vi "Process Incoming Messages by PDU F.vi"(8 "error in":errorcluster, 10 "CAN Frame":T1 {"payload" format="%x"; "timestamp" format="%<%.7X\n%x>T"; "type" items=["CAN Data"=0, "CAN Remote"=1, "CAN Bus Error"=2, "J1939 Data"=192, "Delay"=224, "Log Trigger"=225, "Start Trigger"=226]; "identifier" format="%x"}, 11 "internal data":T3={"J1939 XNET Settings"={"XNET Database"="", "XNET Cluster"="", "CAN port"="", "Baud rate [Bd]"=0, "J1939 Network Address"=0, "Name"=0, "Termination"=0}, "j1939 queues"={"Processed Outgoing"=refnum, "Process Outgoing"=refnum, "stop notifier"=refnum, "error queue"=refnum, "active dtc"=refnum, "processed inc"=refnum}, "fgv references"={"BAM Buffer"=refnum, "CM Buffer"=refnum, "CM Gen"=refnum, "BAM Gen"=refnum, "Address Claims"=refnum, "RQST"=refnum, "scaling lut"=refnum, "data lut"=refnum, "cyclic scheduler"=refnum}, "frame in"="", "frame out"="", "timing"={"tb to j1939 queue timeout"=100, "j1939 to tb queue timeout"=100, "dtc loop period (ms)"=100, "CAN in loop period (ms)"=100, "process incoming queue timeout (ms)"=100, "Outgoing Write Decimation"=0, "process outgoing loop rate (ms)"=0, "periodic outgoing queue timeout (ms)"=10, "CAN out queue timeout (ms)"=100}}) -> (0 "error out":errorcluster)   [LabVIEW 2013, in "J1939.lvlib"]
uses:
  J1939.lvlib
  API Types/Internal Data.ctl
  API Types/XNET Settings.ctl
  API Types/Setup Information Cluster.ctl
  API Types/CAN Outgoing Message Cluster.ctl
  API Types/Convert DTCs Cluster.ctl
  <vilib>/xnet/xnet.llb/XNET Frame CAN.ctl
  <vilib>/xnet/xnet.llb/XNET Frame Type CAN.ctl
  TP/TP List References.ctl
  BAM/BAM Buffer Connections List_Ref.ctl
  Connection Mode/Connection Mode Generation Connection Ref.ctl
  BAM/BAM Generation Connections List_Ref.ctl
  LUTs/J1939 Address Table Reference.ctl
  RQST/RQST Lookup Table Reference.ctl
  LUTs/J1939 Conversion Lookup Table Reference.ctl
  LUTs/J1939 Data Lookup Table Reference.ctl
  LUTs/Cyclic Frame Scheduler Lut Reference.ctl
  Configuration/TypeDefs/timing configuration.ctl
  API Types/PGN Fields Cluster.ctl
  TP/TP Connections List State.ctl
  Connection Mode/Connection Mode Buffer Create New TP Connection State.ctl
  LUTs/J1939 Address Lookup Table Action.ctl
  LUTs/J1939 Address Lookup Table Data.ctl
  Frame Conversion/Convert CAN Arb ID to J1939 ID.vi
  Frame Conversion/Convert J1939 ID to CAN Arb ID.vi
  Frame Conversion/Convert CAN Data (U32) to U8.vi
  Common Messages/J1939 Message Acknowledgement.vi
  Buffer Connections List_Actions.vi
  TP/TP Buffer Search for Connection (No PGN).vi
  TP/TP Buffer Add New Data Packet to Connection.vi
  TP/TP Buffer Convert Connection Info to CAN Frame.vi
  TP/TP Buffer Create New TP Connection.vi
  Common Messages/J1939 Message TP.CM EndofMsgACK.vi
  Common Messages/J1939 Message TP.CM CTS.vi
  Common Messages/J1939 Message TP.Conn Abort.vi
  Connection Mode/Connection Mode Generation Connections List_Actions.vi
  Connection Mode/Connection Mode Generation Search for Connection (Remote Message).vi
  TP/TP Buffer Search for Connection.vi
  Connection Mode/Connection Mode Generation CTS Received.vi
  Conversion Lookup Table Get Conversion Parameter.vi
  LUTs/J1939 Data Lookup Table Get Signals (Range).vi
  Frame Conversion/Convert PGN + SA to J1939 ID.vi
  <vilib>/xnet/xnet.llb/XNET Convert.vi
  <vilib>/xnet/xnet.llb/XNET Convert (Signal to Frame Raw).vi
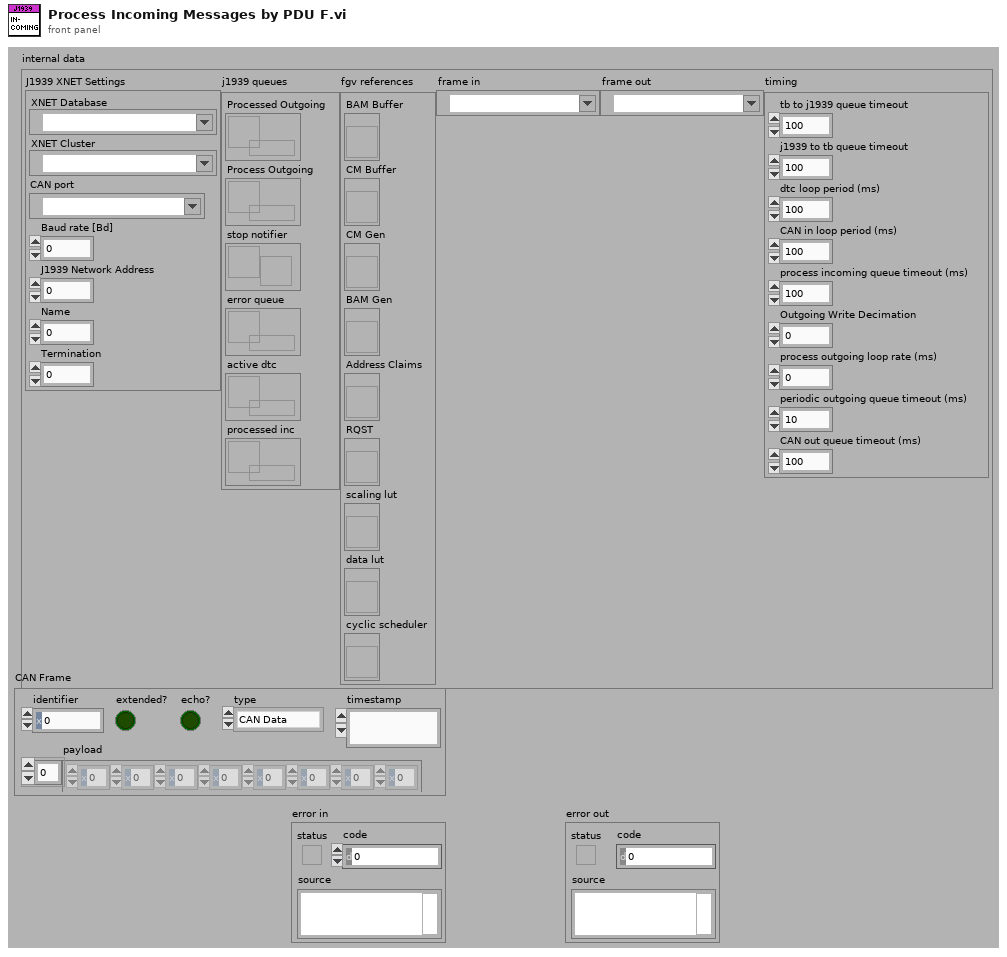
[diagram p1: front panel]
types:
  T1 = typedef "XNET Frame CAN.ctl" = cluster{"timestamp":timestamp, "payload":u8[], "identifier":u32, "type":T2, "extended?":bool, "echo?":bool}
  T2 = typedef "XNET Frame Type CAN.ctl" = u8
  T3 = typedef "J1939.lvlib/Internal Data.ctl" = cluster{"J1939 XNET Settings":T4, "j1939 queues":T5, "fgv references":T6, "frame in":refnum<k21>, "frame out":refnum<k21>, "timing":T15}
  T4 = typedef "J1939.lvlib/XNET settings.ctl" = cluster{"XNET Database":refnum<k21>, "XNET Cluster":refnum<k21>, "CAN port":refnum<k21>, "Baud rate [Bd]":u32, "J1939 Network Address":u8, "Name":u64, "Termination":u32}
  T5 = typedef "J1939.lvlib/Setup Information Cluster.ctl" = cluster{"Processed Outgoing":refnum<queue>, "Process Outgoing":refnum<queue>, "stop notifier":refnum<notifier>, "error queue":refnum<queue>, "active dtc":refnum<queue>, "processed inc":refnum<queue>}
  T6 = typedef "J1939.lvlib/TP List References.ctl" = cluster{"BAM Buffer":T7, "CM Buffer":T7, "CM Gen":T8, "BAM Gen":T9, "Address Claims":T10, "RQST":T11, "scaling lut":T12, "data lut":T13, "cyclic scheduler":T14}
  T7 = typedef "J1939.lvlib/BAM Buffer Connections List_Ref.ctl" = refnum<vi>
  T8 = typedef "J1939.lvlib/Connection Mode Generation Connection Ref.ctl" = refnum<vi>
  T9 = typedef "J1939.lvlib/BAM Generation Connections List_Ref.ctl" = refnum<vi>
  T10 = typedef "J1939.lvlib/J1939 Address Table Reference.ctl" = refnum<vi>
  T11 = typedef "J1939.lvlib/RQST Lookup Table Reference.ctl" = refnum<vi>
  T12 = typedef "J1939.lvlib/J1939 Conversion Lookup Table Reference.ctl" = refnum<vi>
  T13 = typedef "J1939.lvlib/J1939 Data Lookup Table Reference.ctl" = refnum<vi>
  T14 = typedef "J1939.lvlib/cyclic frame scheduler lut reference.ctl" = refnum<vi>
  T15 = typedef "J1939.lvlib/timing configuration.ctl" = cluster{"tb to j1939 queue timeout":i32, "j1939 to tb queue timeout":i32, "dtc loop period (ms)":i32, "CAN in loop period (ms)":i32, "process incoming queue timeout (ms)":i32, "Outgoing Write Decimation":u32, "process outgoing loop rate (ms)":i32, "periodic outgoing queue timeout (ms)":i32, "CAN out queue timeout (ms)":i32}
  T16 = typedef "J1939.lvlib/Message Types.ctl" = enum8{"PDU 1", "RQST2", "XFER", "ACKM", "RQST", "TP.DT - RTS/CTS", "TP.DT - BAM", "TP.CM - RTS", "TP.CM - CTS", "TP.CM - EndofMsgACK", "TP.CM - BAM", "TP.CM - Abort", "TP.CM - Error", "ACL", "Proprietary A", "PDU 2", "Proprietary B", "Error"}
  T17 = typedef "J1939.lvlib/PGN Fields Cluster.ctl" = cluster{"Reserved Bit":u8, "Data page":u8, "PDU Format":u8, "PDU Specific":u8}
  T18 = typedef "J1939.lvlib/CAN Outgoing Message Cluster.ctl" = cluster{"Identifier":u32, "Data":u8[]}
  T19 = typedef "J1939.lvlib/TP Connections List State.ctl" = enum16{"Add", "Update", "Get", "Remove", "Initialize"}
  T20 = typedef "J1939.lvlib/Connection Mode Buffer Create New TP Connection State.ctl" = enum8{"Find Connection", "Create Connection", "Create CTS Frame", "Abort New Connection"}
  T21 = typedef "J1939.lvlib/J1939 Address Lookup Table Data.ctl" = cluster{"Name":u8[], "Address":u8}
  T22 = typedef "J1939.lvlib/J1939 Address Lookup Table Action.ctl" = enum16{"Initialize", "Add", "Get", "Remove", "Get All"}
  T23 = typedef "J1939.lvlib/RQST Lookup Table Cluster.ctl" = cluster{"Response Q":refnum<queue>, "Request PGN":u32}
  T24 = typedef "J1939.lvlib/Convert CAN Data (U8) Cluster.ctl" = cluster{"Byte 1":u8, "Byte 2":u8, "Byte 3":u8, "Byte 4":u8, "Byte 5":u8, "Byte 6":u8, "Byte 7":u8, "Byte 8":u8}
  T25 = typedef "J1939.lvlib/TP Buffer Connection Cluster.ctl" = cluster{"Source Address":u8, "Destination Address":u8, "PGN":u32, "Arb ID":u32, "CAN Conversion Index":u32, "Total Expected Bytes":u16, "Total Expected Packets":u8, "Number of Packets Read":u8, "Start Time":u32, "Packets (U8)":u8[], "Timestamp":timestamp}
  T26 = typedef "J1939.lvlib/Connection Mode Generation Connection Cluster.ctl" = cluster{"Total Packets":u8, "Current Packet to Generate":u8, "Packets":T18[], "Previous Time Stamp":u32, "Total Bytes":u16, "Packet Identifier [PDU S + SA]":u16, "Number of Packets to Generate":u8, "PGN":u32}
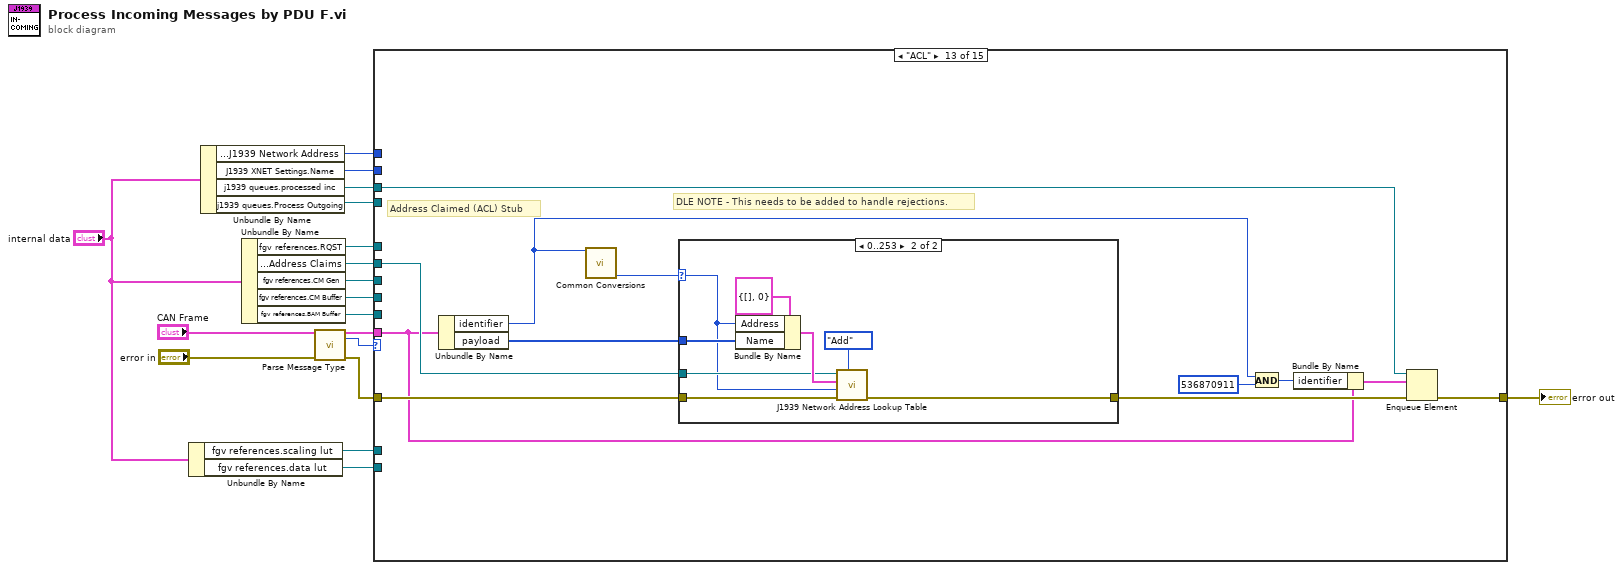
[diagram p0: block diagram]
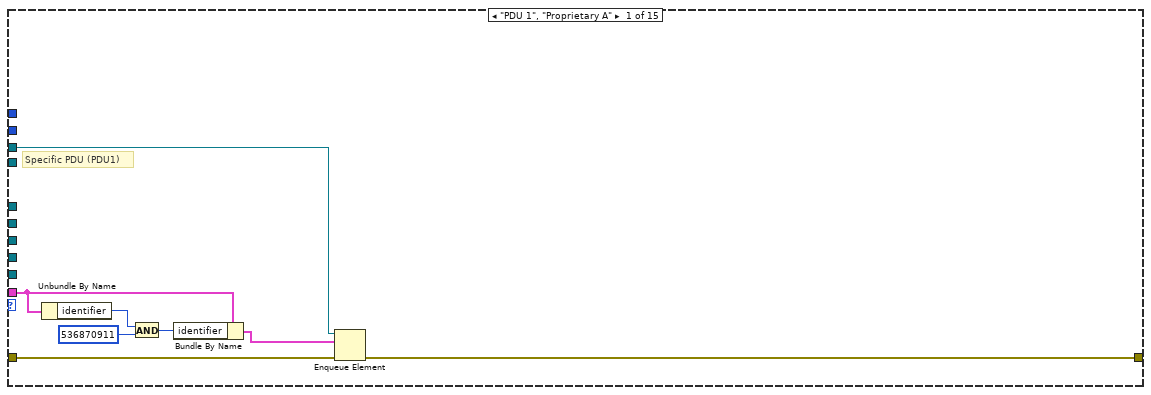
[diagram p2: hidden frame]
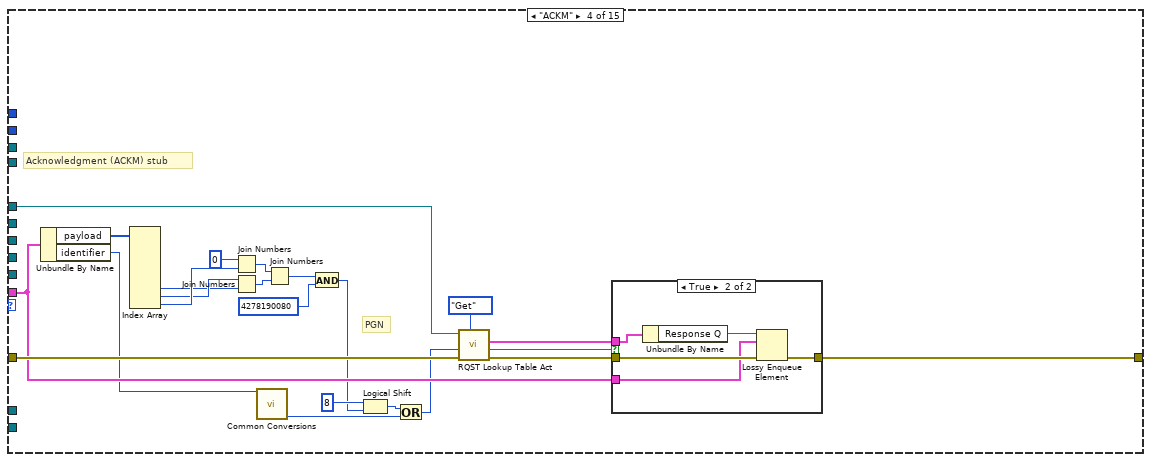
[diagram p5: hidden frame]
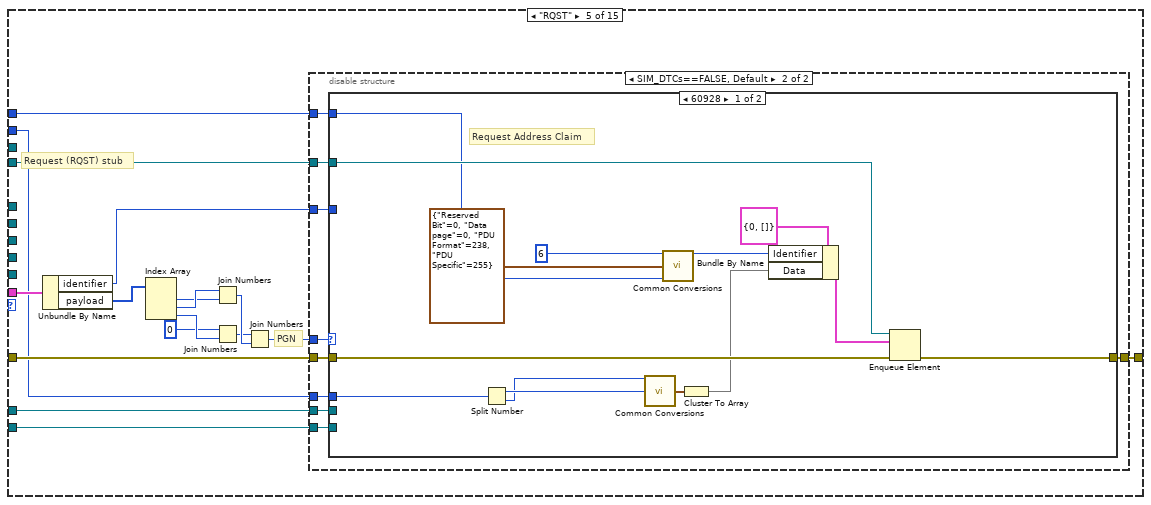
[diagram p7: hidden frame]
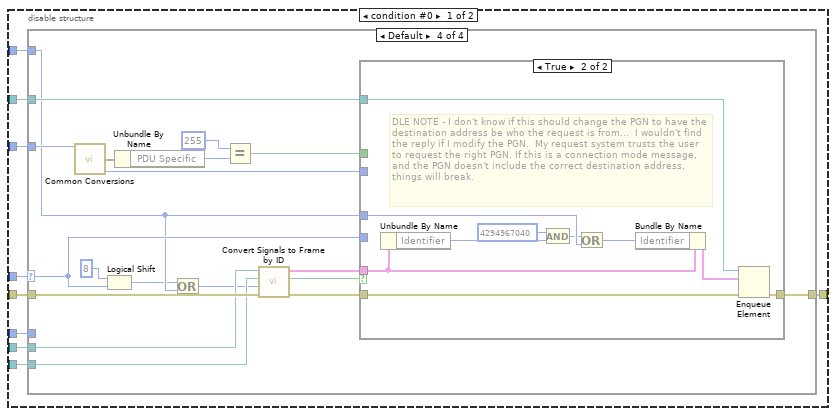
[diagram p8: hidden frame]
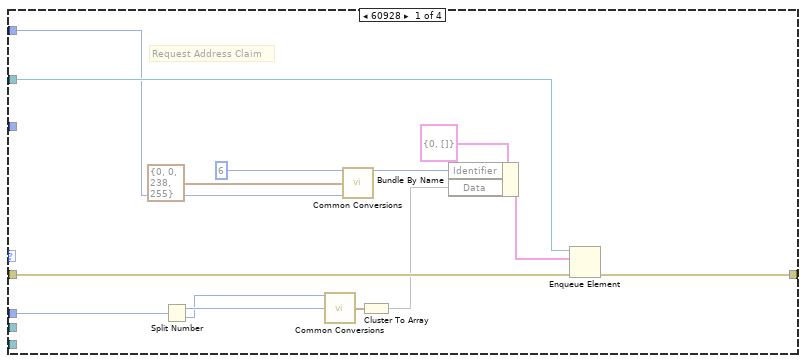
[diagram p9: hidden frame]
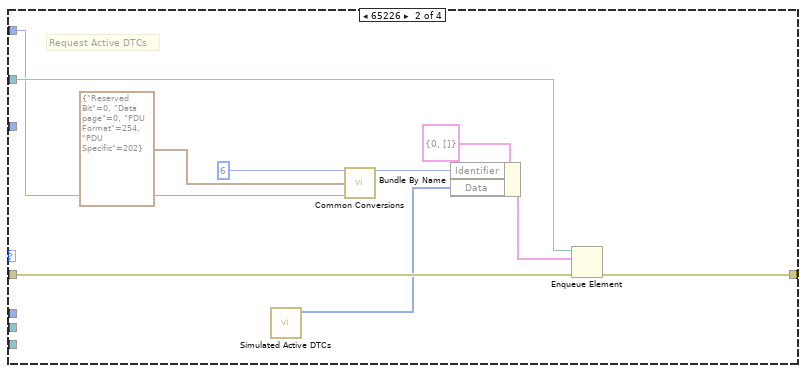
[diagram p10: hidden frame]
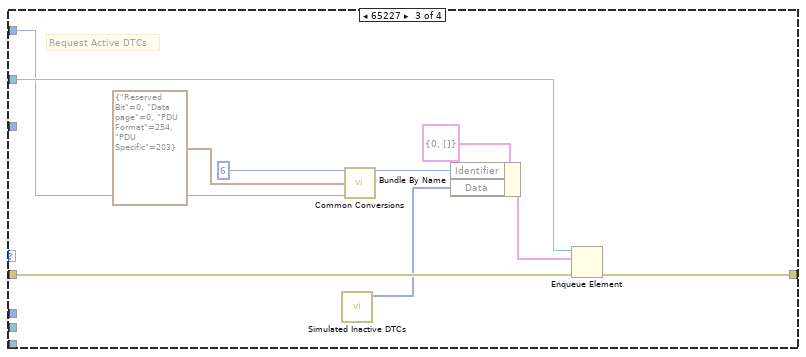
[diagram p11: hidden frame]
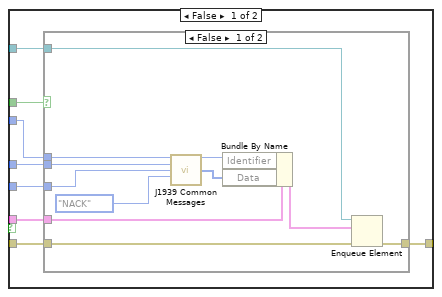
[diagram p12: hidden frame]
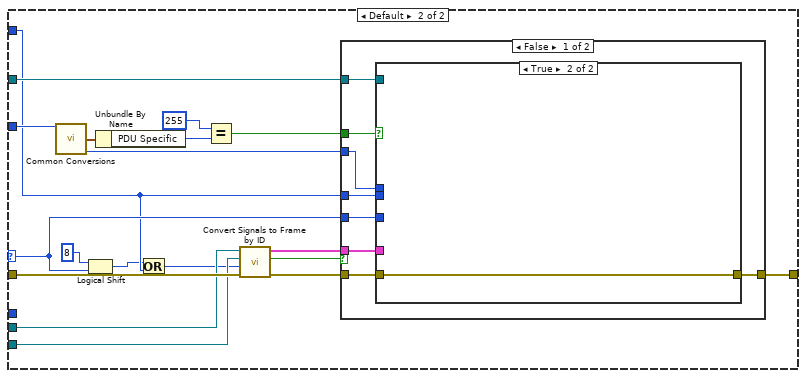
[diagram p14: hidden frame]
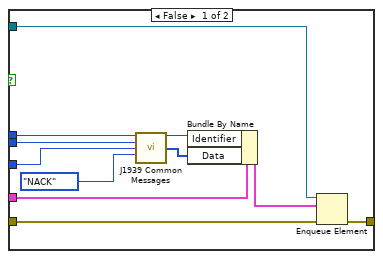
[diagram p15: hidden frame]
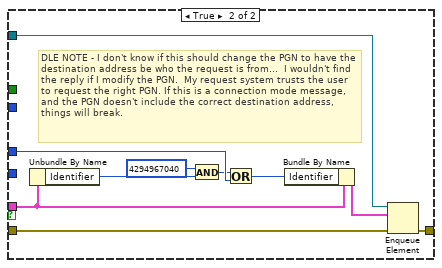
[diagram p16: hidden frame]
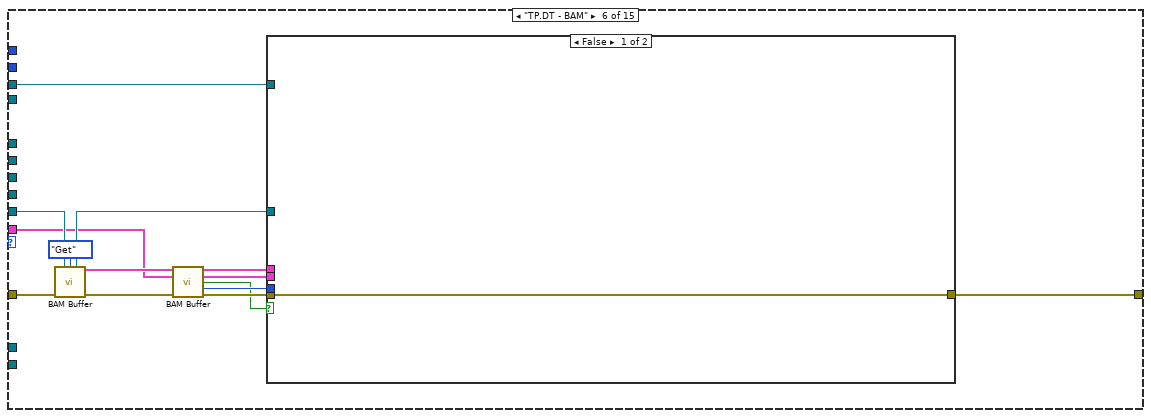
[diagram p17: hidden frame]
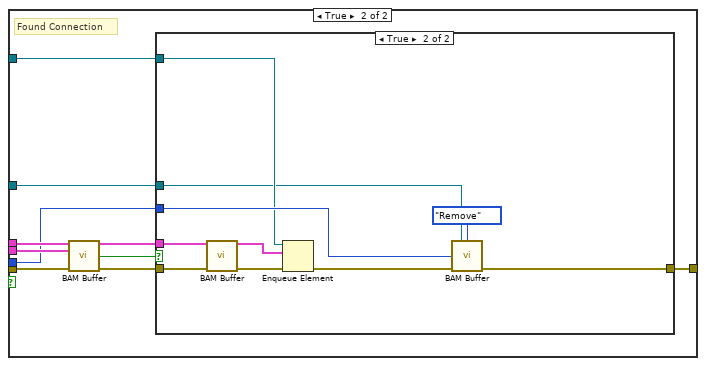
[diagram p18: hidden frame]
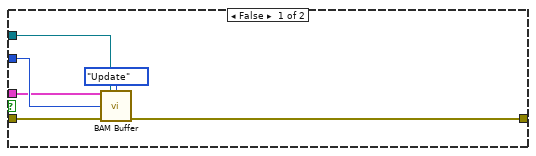
[diagram p19: hidden frame]
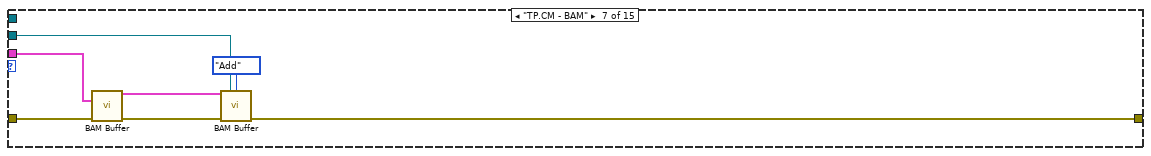
[diagram p20: hidden frame]
diagram:
  n1 = Unbundle By Name("internal data") -> ("fgv references.scaling lut"=w4:T12, "fgv references.data lut"=w3:T13)
  n2 = Unbundle By Name("internal data") -> ("J1939 XNET Settings.J1939 Network Address"=w7:u8, "J1939 XNET Settings.Name"=w8:u64, "j1939 queues.processed inc"=w1:refnum<queue>, "j1939 queues.Process Outgoing"=w13:refnum<queue>)
  n3 = Unbundle By Name("internal data") -> ("fgv references.RQST"=w6:T11, "fgv references.Address Claims"=w9:T10, "fgv references.CM Gen"=w10:T8, "fgv references.CM Buffer"=w11:T7, "fgv references.BAM Buffer"=w12:T7)
  n4 = call "Parse Message Type.vi"("CAN frame"="CAN Frame", "error in"="error in") -> ("CAN frame"=w15:T1, "State"=w14:T16, "error out"=w16:errorcluster)  [unwired: 1 in, 10 out]
  n5 = case shown="\"ACL\"" w14 {
    tunnel: w16 -> [w20 w27 w28 w38 w65 w245 w286 w302 w368 w468 w509 w525 w561 w573 w579]
    tunnel: [w19 w27 w28 w39 w66 w247 w283 w295 w367 w467 w508 w526 w554 w574 w579] -> w18
    tunnel: w15 -> [w24 _ _ w37 w74 w239 w280 w289 w364 w456 w499 w516 w552 w571 _]
    tunnel: w1 -> [w22 _ _ _ _ w242 _ w293 _ _ _ _ w551 w572 _]
    tunnel: w13 -> [_ _ _ _ w64 _ _ w292 w366 _ _ _ _ _ _]
    tunnel: w12 -> [_ _ _ _ _ w241 w281 _ _ _ _ _ _ _ _]
    tunnel: w11 -> [_ _ _ _ _ _ _ w291 w365 w455 _ w519 _ _ _]
    tunnel: w10 -> [_ _ _ _ _ _ _ _ _ w458 w501 w517 _ _ _]
    tunnel: w9 -> [_ _ _ _ _ _ _ _ _ _ _ _ w559 _ _]
    tunnel: w8 -> [_ _ _ _ w63 _ _ _ _ _ _ _ _ _ _]
    tunnel: w7 -> [_ _ _ _ w62 _ _ w288 w363 _ _ _ _ _ _]
    tunnel: w6 -> [_ _ _ w29 _ _ _ _ _ _ _ _ _ _ _]
    tunnel: w4 -> [_ _ _ _ w60 _ _ _ _ _ _ _ _ _ _]
    tunnel: w3 -> [_ _ _ _ w59 _ _ _ _ _ _ _ _ _ _]
    frame "PDU 1", "Proprietary A" {
      # "Specific PDU (PDU1)"
      n6 = Unbundle By Name(w24) -> ("identifier"=w26:u32)
      n7 = And(x=w26, y=u32 536870911) -> (x .and. y?=w23:u32)
      n8 = Bundle By Name(cluster=w24, "identifier"=w23) -> (w21:T1)
      n9 = Enqueue Element(queue=w22, element=w21, error in (no error)=w20) -> (error out=w19:errorcluster)  [unwired: 1 in, 2 out]
    }
    frame "RQST2" {
      # "Request2 (RQST2) Stub"
    }
    frame "XFER" {
      # "Transfer (XFER) Stub"
    }
    frame "ACKM" {
      # "PGN"
      # "Acknowledgment (ACKM) stub"
      n10 = Unbundle By Name(w37) -> ("payload"=w51:u8[], "identifier"=w34:u32)
      n11 = Index Array(array=w51) -> (element #6=w48:u8, element #7=w49:u8, element #8=w50:u8)  [unwired: 8 in, 5 out]
      n12 = Join Numbers(hi=u8 0, lo=w50) -> ((hi.lo)=w47:u16)
      n13 = Join Numbers(hi=w49, lo=w48) -> ((hi.lo)=w46:u16)
      n14 = call-poly "Common Conversions.vi"("Arb ID"=w34) -> ("Source Address"=w33:u8)  [unwired: 11 in, 3 out]
      n15 = Join Numbers(hi=w47, lo=w46) -> ((hi.lo)=w45:u32)
      n16 = And(x=w45, y=u32 4278190080 ("x")) -> (x .and. y?=w32:u32)
      n17 = Logical Shift(y=i8 8, x=w32) -> (x << y=w36:u32)
      n18 = Or(x=w36, y=w33) -> (x .or. y?=w31:u32)
      n19 = call "RQST Lookup Table Act.vi"("Action"=enum16{"Initialize", "Add", "Get", "Remove"}."Get", "error in (no error)"=w38, "ID"=w31, "ref in"=w29) -> ("error out"=w30:errorcluster, "Found?"=w41:bool, "Data"=w40:T23)  [unwired: 5 in]
      n20 = case shown="True" w41 {
        tunnel: w40 -> [_ w56]
        tunnel: w30 -> [w52 w57]
        tunnel: w37 -> [_ w54]
        tunnel: [w52 w53] -> w39
        frame False {
        }
        frame True {
          n21 = Unbundle By Name(w56) -> ("Response Q"=w55:refnum<queue>)
          n22 = Lossy Enqueue Element(queue=w55, element=w54, error in (no error)=w57) -> (error out=w53:errorcluster)  [unwired: 3 out]
        }
      }
    }
    frame "RQST" {
      # "PGN"
      # "Request (RQST) stub"
      n23 = Unbundle By Name(w74) -> ("identifier"=w61:u32, "payload"=w73:u8[])
      n24 = Index Array(array=w73) -> (element #1=w58:u8, element #2=w72:u8, element #3=w71:u8)  [unwired: 3 in]
      n25 = Join Numbers(hi=w72, lo=w58) -> ((hi.lo)=w69:u16)
      n26 = Join Numbers(hi=u8 0, lo=w71) -> ((hi.lo)=w68:u16)
      n27 = Join Numbers(hi=w68, lo=w69) -> ((hi.lo)=w67:u32)
      n28 = disable-structure shown="SIM_DTCs==FALSE, Default" {
        disable-tunnel: w67 -> [w83 w175]
        disable-tunnel: [w82 w174] -> w66
        disable-tunnel: w65 -> [w81 w173]
        disable-tunnel: w64 -> [w80 w172]
        disable-tunnel: w63 -> [w79 w171]
        disable-tunnel: w62 -> [w78 w170]
        disable-tunnel: w61 -> [w77 w169]
        disable-tunnel: w60 -> [w76 w168]
        disable-tunnel: w59 -> [w75 w167]
        frame condition #0 {
          n29 = case shown="Default" w83 {
            selector: w83 -> [_ _ _ w126]
            tunnel: [w92 w99 w109 w127] -> w82
            tunnel: w81 -> [w93 w102 w112 w136]
            tunnel: w80 -> [w90 w101 w111 w128]
            tunnel: w79 -> [w85 _ _ _]
            tunnel: w78 -> [w89 w100 w110 w120]
            tunnel: w77 -> [_ _ _ w129]
            tunnel: w76 -> [_ _ _ w135]
            tunnel: w75 -> [_ _ _ w134]
            frame 60928 {
              # "Request Address Claim"
              n30 = Split Number(x=w85) -> (hi(x)=w87:u32, lo(x)=w86:u32)
              n31 = call-poly "Common Conversions.vi"("Data 0-3"=w86, "Data 4-7"=w87) -> ("Byte Cluster"=w88:T24)  [unwired: 13 in]
              n32 = call-poly "Common Conversions.vi"("Priority"=u8 6, "PGN Fields"=T17 {"Reserved Bit"=0, "Data page"=0, "PDU Format"=238, "PDU Specific"=255}, "Source Address"=w89) -> ("ID"=w95:u32)  [unwired: 2 in, 10 out]
              n33 = Cluster To Array(cluster=w88) -> (array=w84:u8[])
              n34 = Bundle By Name(cluster=T18 {"Identifier"=0, "Data"=[]} ("Data to Send"), "Identifier"=w95, "Data"=w84) -> (w91:T18)
              n35 = Enqueue Element(queue=w90, element=w91, error in (no error)=w93) -> (error out=w92:errorcluster)  [unwired: 1 in, 2 out]
            }
            frame 65226 {
              # "Request Active DTCs"
              n36 = call "Simulated Active DTCs.vi"() -> ("payload"=w98:u8[])  [unwired: 11 in]
              n37 = call-poly "Common Conversions.vi"("Priority"=u8 6, "PGN Fields"=T17 {"Reserved Bit"=0, "Data page"=0, "PDU Format"=254, "PDU Specific"=202}, "Source Address"=w100) -> ("ID"=w105:u32)  [unwired: 2 in, 10 out]
              n38 = Bundle By Name(cluster=T18 {"Identifier"=0, "Data"=[]} ("Data to Send"), "Identifier"=w105, "Data"=w98) -> (w103:T18)
              n39 = Enqueue Element(queue=w101, element=w103, error in (no error)=w102) -> (error out=w99:errorcluster)  [unwired: 1 in, 2 out]
            }
            frame 65227 {
              # "Request Active DTCs"
              n40 = call "Simulated Inactive DTCs.vi"() -> ("payload"=w108:u8[])  [unwired: 11 in]
              n41 = call-poly "Common Conversions.vi"("Priority"=u8 6, "PGN Fields"=T17 {"Reserved Bit"=0, "Data page"=0, "PDU Format"=254, "PDU Specific"=203}, "Source Address"=w110) -> ("ID"=w115:u32)  [unwired: 2 in, 10 out]
              n42 = Bundle By Name(cluster=T18 {"Identifier"=0, "Data"=[]} ("Data to Send"), "Identifier"=w115, "Data"=w108) -> (w113:T18)
              n43 = Enqueue Element(queue=w111, element=w113, error in (no error)=w112) -> (error out=w109:errorcluster)  [unwired: 1 in, 2 out]
            }
            frame Default {
              n44 = call-poly "Common Conversions.vi"("Arb ID"=w129) -> ("PGN Fields"=w125:T17, "Source Address"=w121:u8)  [unwired: 11 in, 2 out]
              n45 = Logical Shift(y=i8 8, x=w126) -> (x << y=w119:u32)
              n46 = Unbundle By Name(w125) -> ("PDU Specific"=w123:u8)
              n47 = Or(x=w119, y=w120) -> (x .or. y?=w118:u32)
              n48 = Equal?(x=u8 255 ("y"), y=w123) -> (x = y?=w122:bool)
              n49 = call "Convert Signals to Frame by ID.vi"("error in (no error)"=w136, "ID"=w118, "Data Ref"=w134, "Conv Ref"=w135) -> ("error out"=w130:errorcluster, "Found?"=w131:bool, "Frame"=w132:T18)  [unwired: 5 in]
              n50 = case shown="True" w131 {
                tunnel: w132 -> [w138 w166]
                tunnel: w120 -> [w140 w164]
                tunnel: [w143 w159] -> w127
                tunnel: w130 -> [w144 w160]
                tunnel: w121 -> [w141 _]
                tunnel: w128 -> [w142 w161]
                tunnel: w126 -> [w139 _]
                tunnel: w122 -> [w137 _]
                frame False {
                  n51 = case shown="False" w137 {
                    tunnel: w144 -> [w155 w156]
                    tunnel: [w154 w156] -> w143
                    tunnel: w142 -> [w153 _]
                    tunnel: w141 -> [w152 _]
                    tunnel: w140 -> [w151 _]
                    tunnel: w139 -> [w150 _]
                    tunnel: w138 -> [w148 _]
                    frame False {
                      n52 = call-poly "J1939 Common Messages.vi"("Destination Address"=w152, "Source Address"=w151, "PGN"=w150, "Control Byte"=enum8{"ACK", "NACK", "Access Denied"}."NACK") -> ("Arb ID"=w147:u32, "Data"=w146:u8[])  [unwired: 10 in]
                      n53 = Bundle By Name(cluster=w148, "Identifier"=w147, "Data"=w146) -> (w145:T18)
                      n54 = Enqueue Element(queue=w153, element=w145, error in (no error)=w155) -> (error out=w154:errorcluster)  [unwired: 3 out]
                    }
                    frame True {
                    }
                  }
                }
                frame True {
                  # "DLE NOTE - I don't know if this should change the PGN to have the destination address be who the request is from...  I wouldn't find the reply if I modify the PGN.  My request system trusts the user to request the right PGN. If this is a connection mode message, and the PGN doesn't include the correct destination address, things will break."
                  n55 = Unbundle By Name(w166) -> ("Identifier"=w165:u32)
                  n56 = And(x=u32 4294967040 ("y"), y=w165) -> (x .and. y?=w157:u32)
                  n57 = Or(x=w157, y=w164) -> (x .or. y?=w163:u32)
                  n58 = Bundle By Name(cluster=w166, "Identifier"=w163) -> (w162:T18)
                  n59 = Enqueue Element(queue=w161, element=w162, error in (no error)=w160) -> (error out=w159:errorcluster)  [unwired: 3 out]
                }
              }
            }
          }
        }
        frame condition #1 (active) {
          n60 = case shown="60928" w175 {
            selector: w175 -> [_ w198]
            tunnel: [w184 w199] -> w174
            tunnel: w173 -> [w185 w208]
            tunnel: w172 -> [w182 w200]
            tunnel: w171 -> [w177 _]
            tunnel: w170 -> [w181 w192]
            tunnel: w169 -> [_ w201]
            tunnel: w168 -> [_ w207]
            tunnel: w167 -> [_ w206]
            frame 60928 {
              # "Request Address Claim"
              n61 = Split Number(x=w177) -> (hi(x)=w179:u32, lo(x)=w178:u32)
              n62 = call-poly "Common Conversions.vi"("Data 0-3"=w178, "Data 4-7"=w179) -> ("Byte Cluster"=w180:T24)  [unwired: 13 in]
              n63 = call-poly "Common Conversions.vi"("Priority"=u8 6, "PGN Fields"=T17 {"Reserved Bit"=0, "Data page"=0, "PDU Format"=238, "PDU Specific"=255}, "Source Address"=w181) -> ("ID"=w187:u32)  [unwired: 2 in, 10 out]
              n64 = Cluster To Array(cluster=w180) -> (array=w176:u8[])
              n65 = Bundle By Name(cluster=T18 {"Identifier"=0, "Data"=[]} ("Data to Send"), "Identifier"=w187, "Data"=w176) -> (w183:T18)
              n66 = Enqueue Element(queue=w182, element=w183, error in (no error)=w185) -> (error out=w184:errorcluster)  [unwired: 1 in, 2 out]
            }
            frame Default {
              n67 = call-poly "Common Conversions.vi"("Arb ID"=w201) -> ("PGN Fields"=w197:T17, "Source Address"=w193:u8)  [unwired: 11 in, 2 out]
              n68 = Logical Shift(y=i8 8, x=w198) -> (x << y=w191:u32)
              n69 = Unbundle By Name(w197) -> ("PDU Specific"=w195:u8)
              n70 = Or(x=w191, y=w192) -> (x .or. y?=w190:u32)
              n71 = Equal?(x=u8 255 ("y"), y=w195) -> (x = y?=w194:bool)
              n72 = call "Convert Signals to Frame by ID.vi"("error in (no error)"=w208, "ID"=w190, "Data Ref"=w206, "Conv Ref"=w207) -> ("error out"=w202:errorcluster, "Found?"=w203:bool, "Frame"=w204:T18)  [unwired: 5 in]
              n73 = case shown="False" w203 {
                tunnel: w204 -> [w210 w238]
                tunnel: w192 -> [w212 w236]
                tunnel: [w215 w231] -> w199
                tunnel: w202 -> [w216 w232]
                tunnel: w193 -> [w213 _]
                tunnel: w200 -> [w214 w233]
                tunnel: w198 -> [w211 _]
                tunnel: w194 -> [w209 _]
                frame False {
                  n74 = case shown="True" w209 {
                    tunnel: w216 -> [w227 w228]
                    tunnel: [w226 w228] -> w215
                    tunnel: w214 -> [w225 _]
                    tunnel: w213 -> [w224 _]
                    tunnel: w212 -> [w223 _]
                    tunnel: w211 -> [w222 _]
                    tunnel: w210 -> [w220 _]
                    frame False {
                      n75 = call-poly "J1939 Common Messages.vi"("Destination Address"=w224, "Source Address"=w223, "PGN"=w222, "Control Byte"=enum8{"ACK", "NACK", "Access Denied"}."NACK") -> ("Arb ID"=w219:u32, "Data"=w218:u8[])  [unwired: 10 in]
                      n76 = Bundle By Name(cluster=w220, "Identifier"=w219, "Data"=w218) -> (w217:T18)
                      n77 = Enqueue Element(queue=w225, element=w217, error in (no error)=w227) -> (error out=w226:errorcluster)  [unwired: 3 out]
                    }
                    frame True {
                    }
                  }
                }
                frame True {
                  # "DLE NOTE - I don't know if this should change the PGN to have the destination address be who the request is from...  I wouldn't find the reply if I modify the PGN.  My request system trusts the user to request the right PGN. If this is a connection mode message, and the PGN doesn't include the correct destination address, things will break."
                  n78 = Unbundle By Name(w238) -> ("Identifier"=w237:u32)
                  n79 = And(x=u32 4294967040 ("y"), y=w237) -> (x .and. y?=w229:u32)
                  n80 = Or(x=w229, y=w236) -> (x .or. y?=w235:u32)
                  n81 = Bundle By Name(cluster=w238, "Identifier"=w235) -> (w234:T18)
                  n82 = Enqueue Element(queue=w233, element=w234, error in (no error)=w232) -> (error out=w231:errorcluster)  [unwired: 3 out]
                }
              }
            }
          }
        }
      }
    }
    frame "TP.DT - BAM" {
      n83 = call-poly "BAM Buffer.vi"("ref in"=w241, "State"=TP_Connections_List_State."Get", "error in (no error)"=w245) -> ("ref out"=w240:T7, "Connections"=w251:T25[], "error out"=w244:errorcluster)  [unwired: 2 in, 8 out]
      n84 = call-poly "BAM Buffer.vi"("Connecctions"=w251, "CAN frame"=w239, "error in (no error)"=w244) -> ("Connection Cluster Out"=w250:T25, "CAN frame Out"=w249:T1, "Found?"=w243:bool, "Index"=w246:i32, "error out"=w248:errorcluster)  [unwired: 8 out]
      n85 = case shown="False" w243 {
        tunnel: w250 -> [_ w263]
        tunnel: w249 -> [_ w261]
        tunnel: w248 -> [w253 w260]
        tunnel: [w253 w258] -> w247
        tunnel: w246 -> [_ w257]
        tunnel: w242 -> [_ w255]
        tunnel: w240 -> [_ w254]
        frame False {
        }
        frame True {
          # "Found Connection"
          n86 = call-poly "BAM Buffer.vi"("Connection Cluster"=w263, "CAN frame"=w261, "error in (no error)"=w260) -> ("Connection Cluster Out"=w256:T25, "Message Complete?"=w262:bool, "error out"=w259:errorcluster)  [unwired: 10 out]
          n87 = case shown="True" w262 {
            tunnel: w259 -> [w267 w277]
            tunnel: [w266 w275] -> w258
            tunnel: w257 -> [w268 w278]
            tunnel: w256 -> [w264 w276]
            tunnel: w255 -> [_ w272]
            tunnel: w254 -> [w265 w270]
            frame False {
              n88 = call-poly "BAM Buffer.vi"("Connection Cluster"=w264, "ref in"=w265, "State"=TP_Connections_List_State."Update", "index"=w268, "error in (no error)"=w267) -> ("error out"=w266:errorcluster)  [unwired: 7 in, 3 out]
            }
            frame True {
              n89 = call-poly "BAM Buffer.vi"("Connection Cluster"=w276, "error in (no error)"=w277) -> ("CAN frame"=w271:T1, "error out"=w274:errorcluster)  [unwired: 12 out]
              n90 = Enqueue Element(queue=w272, element=w271, error in (no error)=w274) -> (error out=w273:errorcluster)  [unwired: 3 out]
              n91 = call-poly "BAM Buffer.vi"("ref in"=w270, "State"=TP_Connections_List_State."Remove", "index"=w278, "error in (no error)"=w273) -> ("error out"=w275:errorcluster)  [unwired: 1 in, 10 out]
            }
          }
        }
      }
    }
    frame "TP.CM - BAM" {
      n92 = call-poly "BAM Buffer.vi"("CAN frame"=w280, "error in (no error)"=w286) -> ("Connection Cluster Out"=w282:T25, "error out"=w284:errorcluster)  [unwired: 1 in, 11 out]
      n93 = call-poly "BAM Buffer.vi"("Connection Cluster"=w282, "ref in"=w281, "State"=TP_Connections_List_State."Add", "error in (no error)"=w284) -> ("error out"=w283:errorcluster)  [unwired: 1 in, 10 out]
    }
    frame "TP.DT - RTS/CTS" {
      n94 = call-poly "Connnection Mode Buffer.vi"("ref in"=w291, "State"=TP_Connections_List_State."Get", "error in (no error)"=w302) -> ("ref out"=w290:T7, "Connections"=w300:T25[], "error out"=w299:errorcluster)  [unwired: 2 in, 8 out]
      n95 = call-poly "Connnection Mode Buffer.vi"("Connecctions"=w300, "CAN frame"=w289, "error in (no error)"=w299) -> ("Connection Cluster Out"=w297:T25, "CAN frame Out"=w294:T1, "Found?"=w287:bool, "Index"=w296:i32, "error out"=w298:errorcluster)  [unwired: 8 out]
      n96 = case shown="True" w287 {
        tunnel: w298 -> [w303 w316]
        tunnel: w297 -> [_ w315]
        tunnel: w294 -> [_ w314]
        tunnel: w296 -> [_ w311]
        tunnel: [w303 w310] -> w295
        tunnel: w293 -> [_ w309]
        tunnel: w292 -> [_ w306]
        tunnel: w290 -> [_ w305]
        tunnel: w288 -> [_ w304]
        frame False {
        }
        frame True {
          # "Found Connection"
          n97 = call-poly "Connnection Mode Buffer.vi"("Connection Cluster"=w315, "CAN frame"=w314, "error in (no error)"=w316) -> ("Connection Cluster Out"=w312:T25, "Frame Mismatch?"=w307:bool, "Message Complete?"=w308:bool, "error out"=w313:errorcluster)  [unwired: 9 out]
          n98 = case shown="True" w308 {
            tunnel: w313 -> [w322 w341]
            tunnel: [w321 w348] -> w310
            tunnel: w311 -> [w320 w347]
            tunnel: w312 -> [w319 w340]
            tunnel: w309 -> [_ w343]
            tunnel: w307 -> [w318 _]
            tunnel: w306 -> [_ w334]
            tunnel: w305 -> [w317 w333]
            tunnel: w304 -> [_ w331]
            frame False {
              n99 = case shown="False" w318 {
                tunnel: w322 -> [w327 w329]
                tunnel: [w326 w329] -> w321
                tunnel: w320 -> [w325 _]
                tunnel: w319 -> [w324 _]
                tunnel: w317 -> [w323 _]
                frame False {
                  n100 = call-poly "Connnection Mode Buffer.vi"("Connection Cluster"=w324, "ref in"=w323, "State"=TP_Connections_List_State."Update", "index"=w325, "error in (no error)"=w327) -> ("error out"=w326:errorcluster)  [unwired: 10 out]
                }
                frame True {
                }
              }
            }
            frame True {
              n101 = Unbundle By Name(w340) -> ("Source Address"=w339:u8, "Destination Address"=w332:u8, "PGN"=w338:u32, "Total Expected Bytes"=w336:u16, "Number of Packets Read"=w337:u8)
              n102 = Equal?(x=w331, y=w332) -> (x = y?=w330:bool)
              n103 = case shown="True" w330 {
                tunnel: w341 -> [w349 w362]
                tunnel: w339 -> [_ w361]
                tunnel: w338 -> [_ w360]
                tunnel: w337 -> [_ w359]
                tunnel: w336 -> [_ w358]
                tunnel: [w349 w354] -> w335
                tunnel: w334 -> [_ w353]
                tunnel: w332 -> [_ w350]
                frame False {
                }
                frame True {
                  # "Only send if message was intended for our address."
                  n104 = call-poly "Connnection Mode Buffer.vi"("PGN"=w360, "Source Address"=w350, "Destination Address"=w361, "Total Message Size(bytes)"=w358, "Total Number of Packets"=w359, "error in (no error)"=w362) -> ("Arb ID"=w357:u32, "Data"=w356:u8[], "error out"=w355:errorcluster)  [unwired: 7 out]
                  n105 = Bundle(cluster=T18 {"Identifier"=0, "Data"=[]} ("Data to Send"), "Identifier"=w357, "Data"=w356) -> (w351:T18)
                  n106 = Enqueue Element(queue=w353, element=w351, error in (no error)=w355) -> (error out=w354:errorcluster)  [unwired: 3 out]
                }
              }
              n107 = call-poly "Connnection Mode Buffer.vi"("Connection Cluster"=w340, "error in (no error)"=w335) -> ("CAN frame"=w342:T1, "error out"=w345:errorcluster)  [unwired: 12 out]
              n108 = Enqueue Element(queue=w343, element=w342, error in (no error)=w345) -> (error out=w344:errorcluster)  [unwired: 3 out]
              n109 = call-poly "Connnection Mode Buffer.vi"("ref in"=w333, "State"=TP_Connections_List_State."Remove", "index"=w347, "error in (no error)"=w344) -> ("error out"=w348:errorcluster)  [unwired: 1 in, 10 out]
            }
          }
        }
      }
    }
    frame "TP.CM - RTS" {
      n110 = while {
        shift-right: [w374] -> _
        shift-left: Connection_Mode_Buffer_Create_New_TP_Connection_State."Find Connection" ("Action") -> [w381]
        tunnel: w364 -> [w382]
        shift-right: [w379] -> _
        shift-left: _ -> [w373]
        shift-right: [w378] -> _
        shift-left: _ -> [w375]
        shift-right: [w377] -> w367
        shift-left: w368 -> [w380]
        tunnel: w366 -> [w372]
        tunnel: w365 -> [w371]
        tunnel: w363 -> [w370]
        stop <- w376 stop-if-true
        n111 = case shown="\"Abort New Connection\"" w381 {
          selector: w381 -> [_ _ w419 w435]
          tunnel: w382 -> [w393 w405 _ w434]
          tunnel: w380 -> [w392 w407 w422 w433]
          tunnel: [w391 w401 w421 w442] -> w379
          tunnel: [w390 w410 w420 w440] -> w378
          tunnel: [w389 w408 w416 w439] -> w377
          tunnel: [FALSE w397 TRUE TRUE] -> w376
          tunnel: w375 -> [_ w410 w420 w440]
          tunnel: [w385 Connection_Mode_Buffer_Create_New_TP_Connection_State."Create CTS Frame" ("Action") w419 w435] -> w374
          tunnel: w373 -> [_ _ w421 w442]
          tunnel: w372 -> [_ _ w415 w438]
          tunnel: w371 -> [w383 w402 _ _]
          tunnel: w370 -> [_ w399 _ w437]
          frame "Find Connection" {
            n112 = call-poly "Connnection Mode Buffer.vi"("ref in"=w383, "State"=TP_Connections_List_State."Get", "error in (no error)"=w392) -> ("Connections"=w395:T25[], "error out"=w396:errorcluster)  [unwired: 2 in, 9 out]
            n113 = call-poly "Connnection Mode Buffer.vi"("Connecctions"=w395, "CAN frame"=w393, "error in (no error)"=w396) -> ("Connection Cluster Out"=w391:T25, "Found?"=w386:bool, "Index"=w390:i32, "error out"=w389:errorcluster)  [unwired: 9 out]
            n114 = Select(t=Connection_Mode_Buffer_Create_New_TP_Connection_State."Abort New Connection", s=w386, f=Connection_Mode_Buffer_Create_New_TP_Connection_State."Create Connection" ("Action")) -> (s? t:f=w385:T20)
          }
          frame "Create Connection" {
            # "Stop if the intended address wasn't us."
            n115 = call-poly "Connnection Mode Buffer.vi"("CAN frame"=w405, "error in (no error)"=w407) -> ("Connection Cluster Out"=w404:T25, "error out"=w406:errorcluster)  [unwired: 12 out]
            n116 = call-poly "Connnection Mode Buffer.vi"("Connection Cluster"=w404, "ref in"=w402, "State"=TP_Connections_List_State."Add", "error in (no error)"=w406) -> ("Connection Cluster Out"=w401:T25, "error out"=w408:errorcluster)  [unwired: 1 in, 9 out]
            n117 = Unbundle By Name(w401) -> ("Destination Address"=w400:u8)
            n118 = Equal?(x=w399, y=w400) -> (x = y?=w398:bool)
            n119 = Not(x=w398) -> (.not. x?=w397:bool)
          }
          frame "Create CTS Frame" {
            # "Only send if the message was intended for our address."
            n120 = Unbundle By Name(w421) -> ("Source Address"=w427:u8, "Destination Address"=w426:u8, "PGN"=w425:u32, "Total Expected Packets"=w423:u8)
            n121 = call-poly "Connnection Mode Buffer.vi"("PGN"=w425, "Source Address"=w426, "Destination Address"=w427, "Number of Packets to Send"=w423, "Next Packet to Send"=u8 1, "error in (no error)"=w422) -> ("Arb ID"=w414:u32, "Data"=w413:u8[], "error out"=w417:errorcluster)  [unwired: 1 in, 6 out]
            n122 = Bundle(cluster=T18 {"Identifier"=0, "Data"=[]} ("Data to Send"), "Identifier"=w414, "Data"=w413) -> (w411:T18)
            n123 = Enqueue Element(queue=w415, element=w411, error in (no error)=w417) -> (error out=w416:errorcluster)  [unwired: 3 out]
          }
          frame "Abort New Connection" {
            n124 = call-poly "Connnection Mode Buffer.vi"("CAN frame"=w434, "error in (no error)"=w433) -> ("Connection Cluster Out"=w431:T25, "error out"=w432:errorcluster)  [unwired: 12 out]
            n125 = Unbundle By Name(w431) -> ("Source Address"=w430:u8, "Destination Address"=w429:u8, "PGN"=w428:u32)
            n126 = Equal?(x=w437, y=w429) -> (x = y?=w436:bool)
            n127 = case shown="True" w436 {
              tunnel: w432 -> [w443 w454]
              tunnel: [w443 w450] -> w439
              tunnel: w438 -> [_ w447]
              tunnel: w430 -> [_ w446]
              tunnel: w429 -> [_ w445]
              tunnel: w428 -> [_ w444]
              frame False {
              }
              frame True {
                n128 = call-poly "Connnection Mode Buffer.vi"("Destination Address"=w446, "Source Address"=w445, "PGN"=w444, "error in (no error)"=w454) -> ("Arb ID"=w453:u32, "Data"=w452:u8[], "error out"=w451:errorcluster)  [unwired: 2 in, 7 out]
                n129 = Bundle(cluster=T18 {"Identifier"=0, "Data"=[]} ("Data to Send"), "Identifier"=w453, "Data"=w452) -> (w448:T18)
                n130 = Enqueue Element(queue=w447, element=w448, error in (no error)=w451) -> (error out=w450:errorcluster)  [unwired: 3 out]
              }
            }
          }
        }
      }
    }
    frame "TP.CM - CTS" {
      n131 = call-poly "Connection Mode Generation.vi"("ref in"=w458, "State"=TP_Connections_List_State."Get", "error in (no error)"=w468) -> ("ref out"=w457:T8, "Connections"=w459:T26[], "error out"=w460:errorcluster)  [unwired: 2 in, 8 out]
      n132 = call-poly "Connection Mode Generation.vi"("Connections"=w459, "CAN frame"=w456, "error in (no error)"=w460) -> ("Connection Cluster"=w463:T26, "CAN frame out"=w466:T1, "Found?"=w465:bool, "Index"=w464:i32, "error out"=w462:errorcluster)  [unwired: 1 in, 7 out]
      n133 = case shown="False" w465 {
        tunnel: w462 -> [w477 w498]
        tunnel: w463 -> [_ w497]
        tunnel: [w472 w494] -> w467
        tunnel: w464 -> [_ w492]
        tunnel: w466 -> [w475 w491]
        tunnel: w457 -> [_ w490]
        tunnel: w455 -> [w476 _]
        frame False {
          n134 = call-poly "Connnection Mode Buffer.vi"("ref in"=w476, "State"=TP_Connections_List_State."Get", "error in (no error)"=w477) -> ("ref out"=w469:T7, "Connections"=w479:T25[], "error out"=w480:errorcluster)  [unwired: 2 in, 8 out]
          n135 = call-poly "Connnection Mode Buffer.vi"("Connecctions"=w479, "CAN frame"=w475, "error in (no error)"=w480) -> ("Connection Cluster Out"=w470:T25, "Found?"=w474:bool, "Index"=w471:i32, "error out"=w473:errorcluster)  [unwired: 9 out]
          n136 = case shown="True" w474 {
            tunnel: w473 -> [w481 w489]
            tunnel: [w481 w488] -> w472
            tunnel: w471 -> [_ w487]
            tunnel: w470 -> [_ w484]
            tunnel: w469 -> [_ w486]
            frame False {
            }
            frame True {
              n137 = call "Tick Count"() -> ("Tick Count(mSec)"=w482:u32)
              n138 = Bundle By Name(cluster=w484, "Start Time"=w482) -> (w483:T25)
              n139 = call-poly "Connnection Mode Buffer.vi"("Connection Cluster"=w483, "ref in"=w486, "State"=TP_Connections_List_State."Update", "index"=w487, "error in (no error)"=w489) -> ("error out"=w488:errorcluster)  [unwired: 10 out]
            }
          }
        }
        frame True {
          n140 = call-poly "Connection Mode Generation.vi"("Connection Cluster"=w497, "CAN frame"=w491, "error in (no error)"=w498) -> ("Connection Cluster Out"=w496:T26, "error out"=w495:errorcluster)  [unwired: 11 out]
          n141 = call-poly "Connection Mode Generation.vi"("Connection Cluster"=w496, "ref in"=w490, "State"=TP_Connections_List_State."Update", "index"=w492, "error in (no error)"=w495) -> ("error out"=w494:errorcluster)  [unwired: 10 out]
        }
      }
    }
    frame "TP.CM - EndofMsgACK" {
      # "DLE NOTE - Technically, I should wait for this when acquiring a connection mode message from an address other than mine (I generate the message if my address is the one the message is intended for)."
      n142 = call-poly "Connection Mode Generation.vi"("ref in"=w501, "State"=TP_Connections_List_State."Get", "error in (no error)"=w509) -> ("ref out"=w500:T8, "Connections"=w504:T26[], "error out"=w503:errorcluster)  [unwired: 2 in, 8 out]
      n143 = call-poly "Connection Mode Generation.vi"("Connections"=w504, "CAN frame"=w499, "error in (no error)"=w503) -> ("Found?"=w506:bool, "Index"=w507:i32, "error out"=w505:errorcluster)  [unwired: 1 in, 9 out]
      n144 = case shown="True" w506 {
        tunnel: w505 -> [w510 w515]
        tunnel: [w510 w514] -> w508
        tunnel: w507 -> [_ w512]
        tunnel: w500 -> [_ w511]
        frame False {
        }
        frame True {
          n145 = call-poly "Connection Mode Generation.vi"("ref in"=w511, "State"=TP_Connections_List_State."Remove", "index"=w512, "error in (no error)"=w515) -> ("error out"=w514:errorcluster)  [unwired: 1 in, 10 out]
        }
      }
    }
    frame "TP.CM - Abort" {
      n146 = call-poly "Connnection Mode Buffer.vi"("ref in"=w519, "State"=TP_Connections_List_State."Get", "error in (no error)"=w525) -> ("ref out"=w518:T7, "Connections"=w522:T25[], "error out"=w524:errorcluster)  [unwired: 2 in, 8 out]
      n147 = call-poly "Connnection Mode Buffer.vi"("Connecctions"=w522, "CAN frame"=w516, "error in (no error)"=w524) -> ("Found?"=w521:bool, "Index"=w520:i32, "error out"=w527:errorcluster)  [unwired: 1 in, 9 out]
      n148 = case shown="True" w521 {
        tunnel: w527 -> [w537 w549]
        tunnel: [w538 w548] -> w526
        tunnel: w520 -> [_ w546]
        tunnel: w516 -> [w536 _]
        tunnel: w518 -> [_ w545]
        tunnel: w517 -> [w529 _]
        frame False {
          n149 = call-poly "Connection Mode Generation.vi"("ref in"=w529, "State"=TP_Connections_List_State."Get", "error in (no error)"=w537) -> ("ref out"=w528:T8, "Connections"=w532:T26[], "error out"=w531:errorcluster)  [unwired: 2 in, 8 out]
          n150 = call-poly "Connection Mode Generation.vi"("Connections"=w532, "CAN frame"=w536, "error in (no error)"=w531) -> ("Found?"=w534:bool, "Index"=w535:i32, "error out"=w533:errorcluster)  [unwired: 1 in, 9 out]
          n151 = case shown="True" w534 {
            tunnel: w533 -> [w539 w544]
            tunnel: [w539 w543] -> w538
            tunnel: w535 -> [_ w541]
            tunnel: w528 -> [_ w540]
            frame False {
            }
            frame True {
              n152 = call-poly "Connection Mode Generation.vi"("ref in"=w540, "State"=TP_Connections_List_State."Remove", "index"=w541, "error in (no error)"=w544) -> ("error out"=w543:errorcluster)  [unwired: 1 in, 10 out]
            }
          }
        }
        frame True {
          n153 = call-poly "Connnection Mode Buffer.vi"("ref in"=w545, "State"=TP_Connections_List_State."Remove", "index"=w546, "error in (no error)"=w549) -> ("error out"=w548:errorcluster)  [unwired: 1 in, 10 out]
        }
      }
    }
    frame "ACL" {
      # "DLE NOTE - This needs to be added to handle rejections."
      # "Address Claimed (ACL) Stub"
      n154 = Unbundle By Name(w552) -> ("identifier"=w553:u32, "payload"=w560:u8[])
      n155 = call-poly "Common Conversions.vi"("Arb ID"=w553) -> ("Source Address"=w550:u8)  [unwired: 11 in, 3 out]
      n156 = case shown="0..253" w550 {
        selector: w550 -> [_ w564]
        tunnel: w561 -> [w562 w569]
        tunnel: [w562 w563] -> w555
        tunnel: w560 -> [_ w567]
        tunnel: w559 -> [_ w565]
        frame Default {
        }
        frame 0..253 {
          n157 = Bundle By Name(cluster=T21 {"Name"=[], "Address"=0} ("Data"), "Address"=w564, "Name"=w567) -> (w566:T21)
          n158 = call "J1939 Network Address Lookup Table.vi"("Action"=J1939_Address_Lookup_Table_Action."Add", "error in (no error)"=w569, "Address"=w564, "Data"=w566, "ref in"=w565) -> ("error out"=w563:errorcluster)  [unwired: 3 in, 3 out]
        }
      }
      n159 = And(x=w553, y=u32 536870911) -> (x .and. y?=w556:u32)
      n160 = Bundle By Name(cluster=w552, "identifier"=w556) -> (w557:T1)
      n161 = Enqueue Element(queue=w551, element=w557, error in (no error)=w555) -> (error out=w554:errorcluster)  [unwired: 3 out]
    }
    frame "PDU 2", "Proprietary B" {
      # "Global PDUs (PDU2)"
      n162 = Unbundle By Name(w571) -> ("identifier"=w578:u32)
      n163 = And(x=w578, y=u32 536870911) -> (x .and. y?=w575:u32)
      n164 = Bundle By Name(cluster=w571, "identifier"=w575) -> (w576:T1)
      n165 = Enqueue Element(queue=w572, element=w576, error in (no error)=w573) -> (error out=w574:errorcluster)  [unwired: 3 out]
    }
    frame "TP.CM - Error", "Error" {
      # "Proprietary B Stub"
    }
  }
  "error out" <- w18
